vi "Recive Data.vi"(8 "error in (no error)":errorcluster, 11 "RP Transceiver in":refnum<class "RP Transceiver.lvclass">) -> (0 "error out":errorcluster, 2 "Data out":i32[](array[numeric]), 3 "RP Transceiver out":refnum<class "RP Transceiver.lvclass">)   [LabVIEW 2015, in "RP Transceiver.lvclass"]
uses:
  RP Transceiver.lvclass
  RP Transceiver.lvclass/RP Transceiver.ctl
  RP Communicator/RP Communicator.lvclass
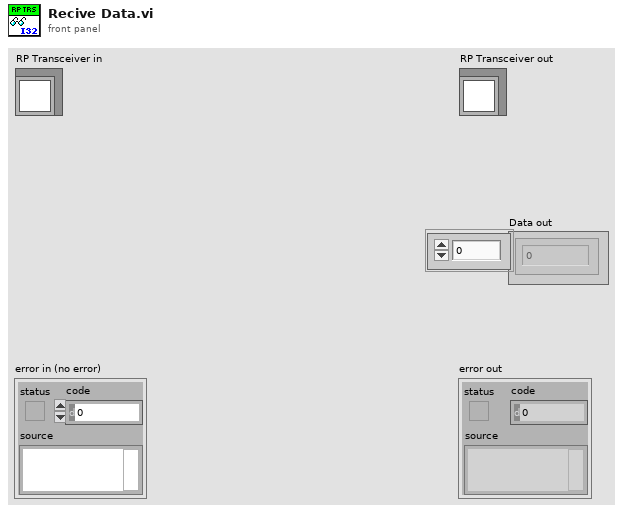
[diagram p1: front panel]
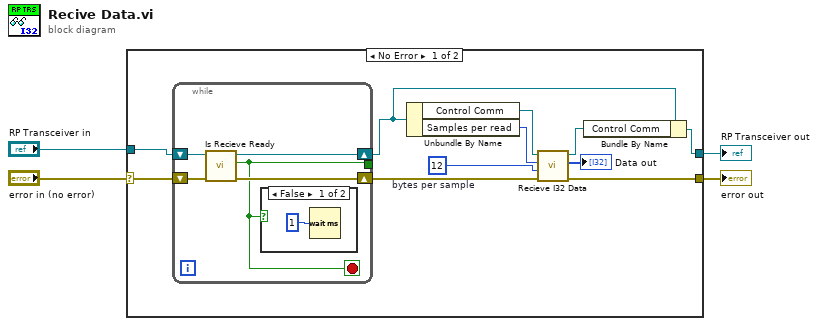
[diagram p0: block diagram]
diagram:
  n1 = case shown="No Error" "error in (no error)" {
    selector: "error in (no error)" -> [w8 w23]
    tunnel: [w9 w23] -> w3
    tunnel: [w10 w22] -> w1
    tunnel: "RP Transceiver in" -> [w5 w22]
    frame No Error {
      w13 = 12  # bytes per sample
      n2 = while {
        shift-right: [w18] -> w7
        shift-left: w8 -> [w19]
        shift-right: [w17] -> w6
        shift-left: w5 -> [w20]
        tunnel: [w16] -> _
        stop <- w16 stop-if-true
        n3 = call-dynamic "Is Recieve Ready.vi"("error in (no error)"=w19, "RP Lockin in"=w20) -> ("error out"=w18:errorcluster, "Recieve Ready"=w16:bool, "RP Lockin out"=w17:refnum<class "RP Transceiver.lvclass">)  [unwired: 7 in]
        n4 = case shown="False" w16 {
          frame False {
            n5 = Wait (ms)(milliseconds to wait=u32 1) -> ()  [unwired: 1 out]
          }
          frame True {
          }
        }
      }
      n6 = Unbundle By Name(w6) -> ("Control Comm"=w11:refnum<class "RP Communicator.lvclass">, "Samples per read"=w12:i32)
      n7 = call-dynamic "Recieve I32 Data.vi"("error in (no error)"=w7, "bytes per sample"=w13, "Samples per read"=w12, "RP Communicator in"=w11) -> ("error out"=w9:errorcluster, "Data out"=→"Data out":i32[], "RP Communicator out"=w14:refnum<class "RP Communicator.lvclass">)  [unwired: 5 in]
      n8 = Bundle By Name(cluster=w6, "Control Comm"=w14) -> (w10:refnum<class "RP Transceiver.lvclass">)
    }
    frame Error {
    }
  }
  "error out" <- w3
  "RP Transceiver out" <- w1
